vi "Build Measurement.vi"() -> ()   [LabVIEW 2021]
uses:
  <vilib>/Utility/miscctls.llb/LVRowAndColumnTypeDef.ctl
  _Measurement Builder/Measurement Builder/Queue Driver/controls/Queue Operations.ctl
  _Measurement Builder/Measurement Builder/controls/Config File Operations.ctl
  _Measurement Builder/Measurement Builder/controls/Data Holder.ctl
  <vilib>/Utility/miscctls.llb/LVPoint32TypeDef.ctl
  _Measurement Builder/Measurement Builder/controls/Build Spec Details.ctl
  <vilib>/AppBuilder/AB_API_Simple/Get Build Specification Version (path).vi
  _Measurement Builder/Measurement Builder/Queue Driver/Queue Driver.lvlib
  _Measurement Builder/Measurement Builder/Measurement Builder.lvlib
  _Measurement Builder/Measurement Builder/Dictionary/Dictionary.lvlib
  <vilib>/AppBuilder/AB_API_Simple/NI_App_Builder_API.lvlib
panel:
  out "error out":errorcluster
  out "Tab Control":T1(tab)
  in  "Open Directory":bool
  in  "Feed Path":path
  out "Warning":bool=TRUE caption="Feed Path cannot be empty/invalid"
  in  "Next to select":bool
  in  "Build Package":bool
  in  "Project":path caption="LabVIEW Project Path"
  in  "Feed":T2(radio)
  in  "Back 1":bool
  in  "Populate Package":bool
  in  "Select All":bool
  out "Measurement List":i32(listbox)=-1 caption="Select the Measurements to build the package"
  out "Selection warning":string="Selected Project doesn't have EXE build spec"
  out "Maintainer Warning":string
  in  "Settings Page":enum32{"Page 1", "Page 2"}(tab)
  in  "Maintainer Email ID":string="sabthagiri@ni.com"
  in  "Architecture":string(combo)="1"
  in  "Maintainer":string="NI"
  in  "Back 2":bool
  in  "Start Build":bool
  in  "Package List":i32[](listbox) caption="Edit the Package Name and Version"
  in  "Settings":bool
  in  "Progres Bar":i32(slide)=9 caption="Creating Distribution..." scale=0.0..100.0
  in  "Start Next":bool
  in  "Log":bool[](array[boolean])=[TRUE, TRUE]
  in  "Build Status":i32(listbox)=-1
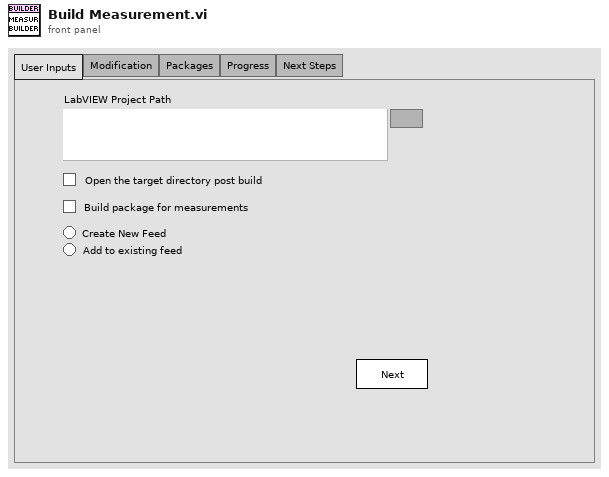
[diagram p1: front panel]
types:
  T1 = enum32{"User Inputs", "Modification", "Packages", "Progress", "Next Steps"}
  T2 = enum32{"No Selection", "CreateFeed", "AddtoFeed"}
  T3 = typedef "Queue Driver.lvlib/Queue Operations.ctl" = enum16{"Create Q", "Enqueue", "Enqueue N", "Dequeue", "Flush", "Release"}
  T4 = typedef "LVRowAndColumnTypeDef.ctl" = cluster{"Row":i32, "Column":i32}
  T5 = enum8{"Enabled", "Disabled", "Disabled and Grayed Out"}
  T6 = typedef "Measurement Builder.lvlib/Config File Operations.ctl" = enum16{"Read", "Write"}
  T7 = typedef "Measurement Builder.lvlib/Data Holder.ctl" = cluster{"Next Clicked?":bool, "MosueDown Coords":T8, "Build Spec":T9[], "No of Meas":i32, "No. of Selected Meas":i32, "Selected Meas":T9[], "Package Details":string[][], "Build Packge?":bool, "Packages Path":path, "Feed":enum32{"No Selection", "CreateFeed", "AddtoFeed"}, "Feed Path":path, "Valid Inputs?":bool, "Feed Old":enum32{"No Selection", "CreateFeed", "AddtoFeed"}, "Status":string[], "Open Directory?":bool}
  T8 = typedef "LVPoint32TypeDef.ctl" = cluster{"Horizontal":i32, "Vertical":i32}
  T9 = typedef "Measurement Builder.lvlib/Build Spec Details.ctl" = cluster{"EXE Name":string, "Target path":path, "Has PPL?":bool, "PPL Name":string}
  T10 = typedef "NI_App_Builder_API.lvlib/Build Specification Version.ctl" = cluster{"Major":u16, "Minor":u16, "Fix":u16, "Build":u16}
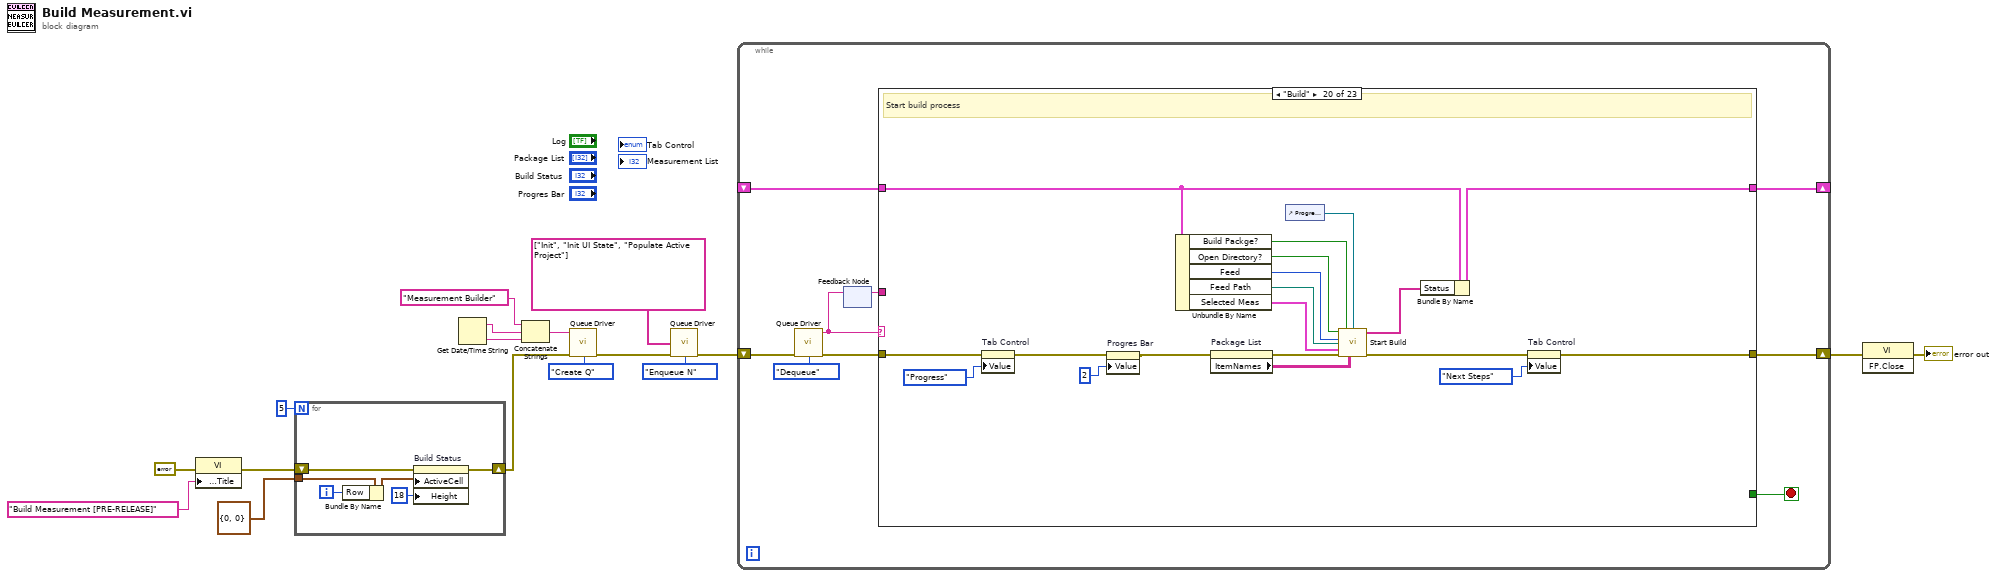
[diagram p0: block diagram]
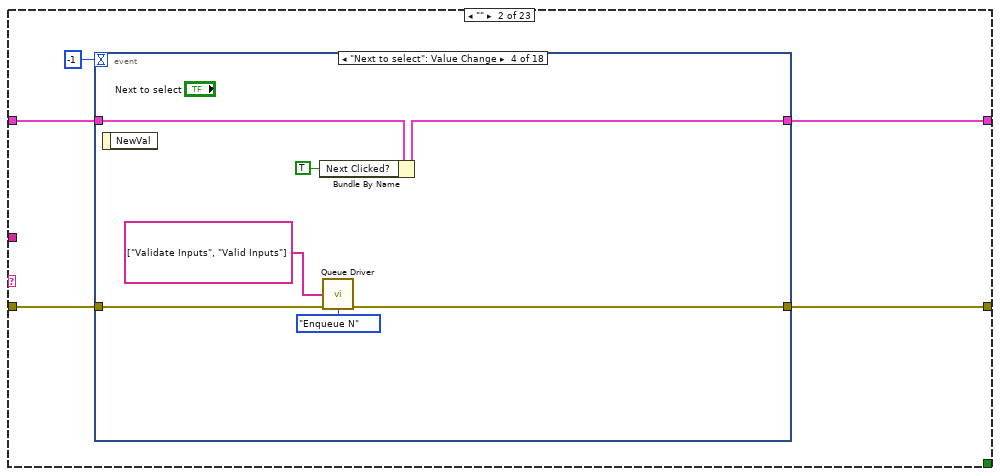
[diagram p3: hidden frame]
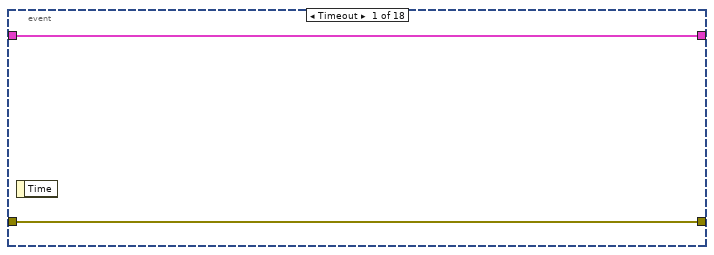
[diagram p4: hidden frame]
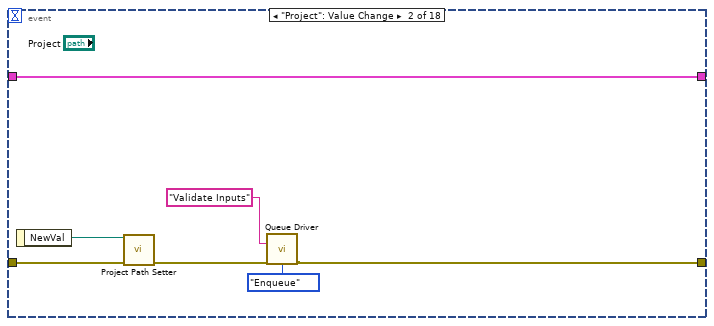
[diagram p5: hidden frame]
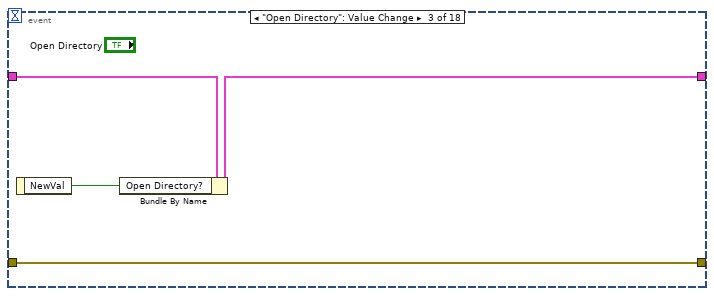
[diagram p6: hidden frame]
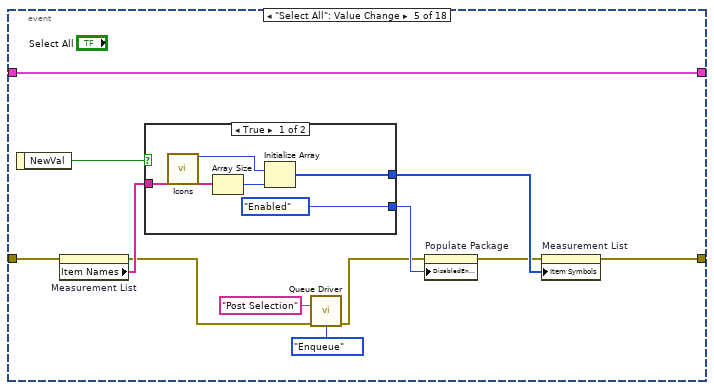
[diagram p7: hidden frame]
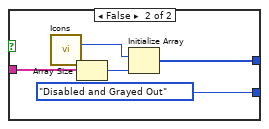
[diagram p8: hidden frame]
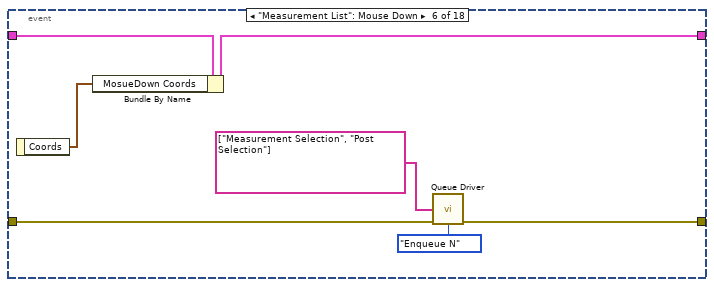
[diagram p9: hidden frame]
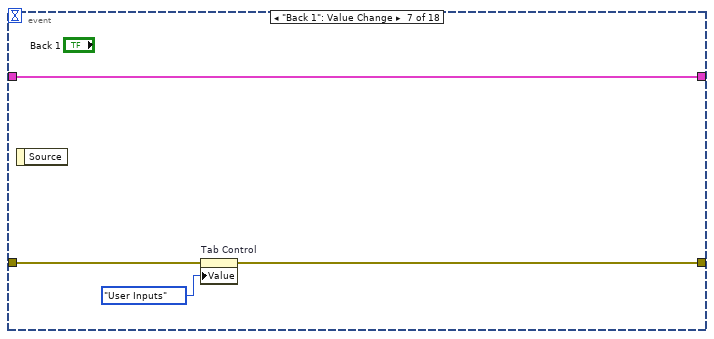
[diagram p10: hidden frame]
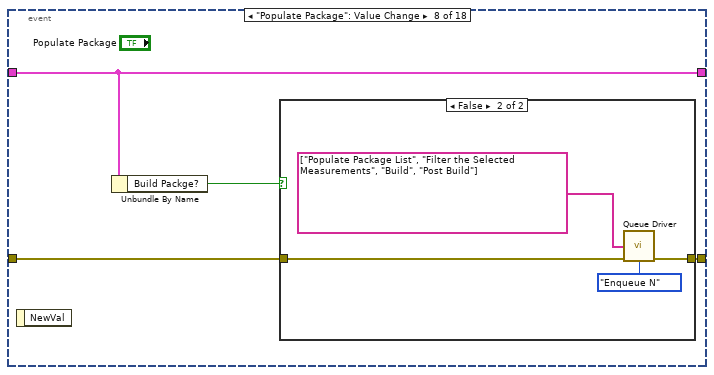
[diagram p11: hidden frame]
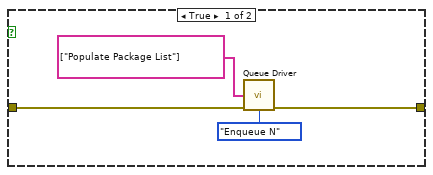
[diagram p12: hidden frame]
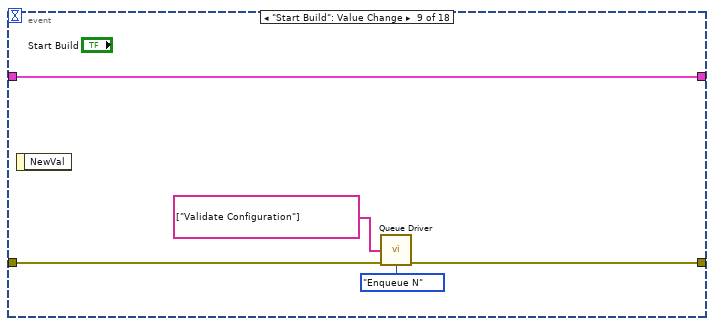
[diagram p13: hidden frame]
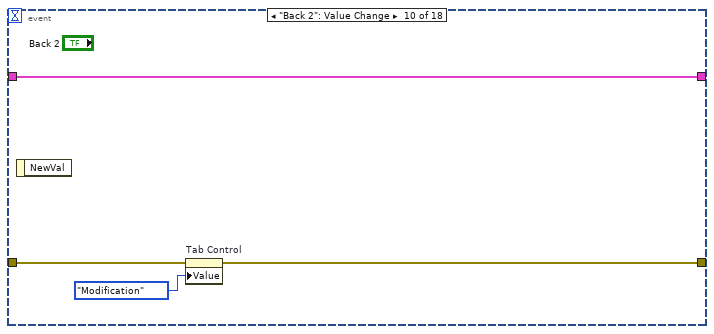
[diagram p14: hidden frame]
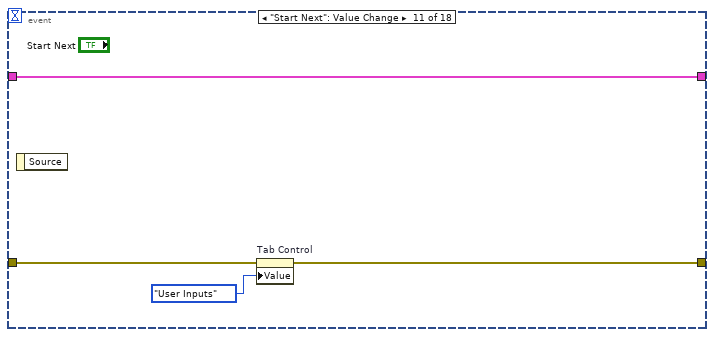
[diagram p15: hidden frame]
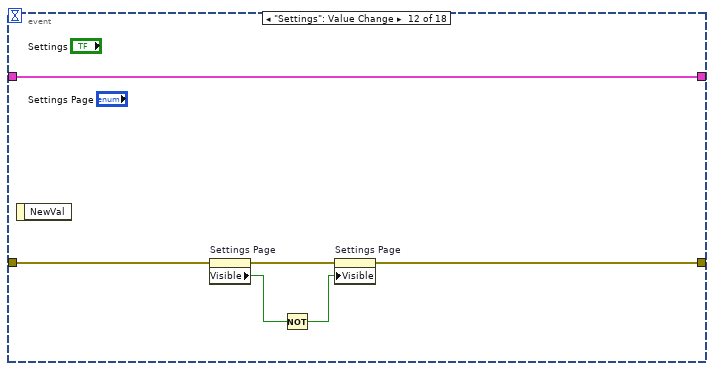
[diagram p16: hidden frame]
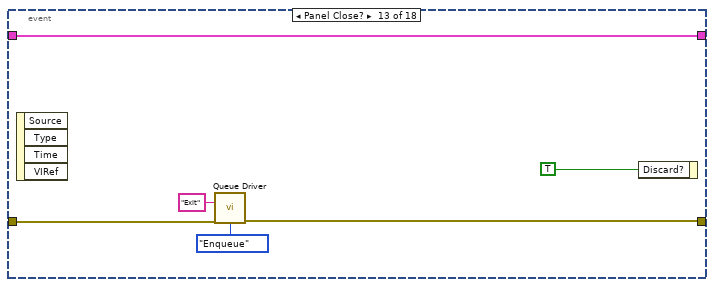
[diagram p17: hidden frame]
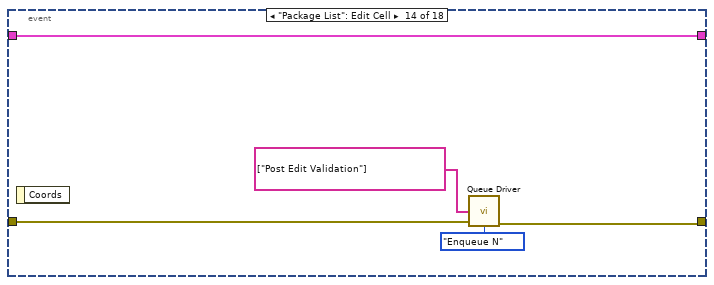
[diagram p18: hidden frame]
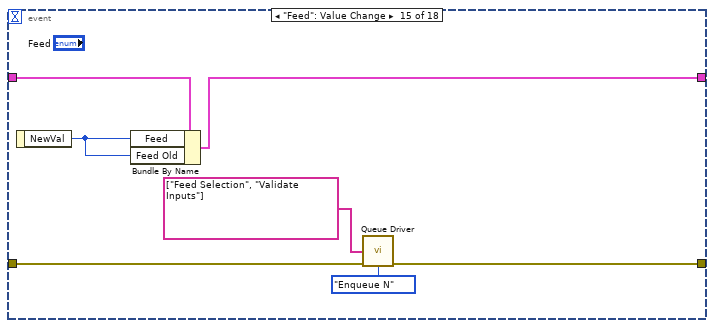
[diagram p19: hidden frame]
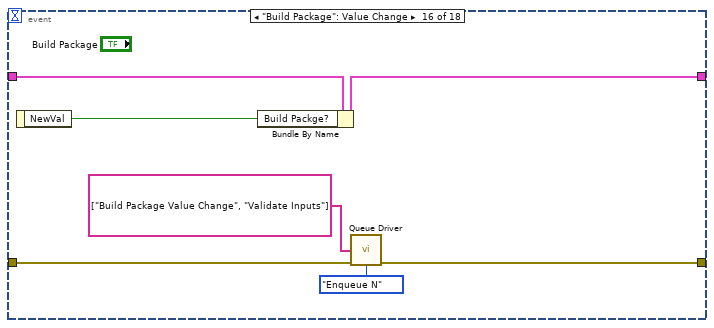
[diagram p20: hidden frame]
diagram:
  n1 = property class="VI"(error in=errorcluster {"status"=FALSE, "code"=0, "source"=""} ("error in (no error)"), "Front Panel.Title"="Build Measurement [PRE-RELEASE]" ("Front Panel Window:Title")) -> (error out=w3:errorcluster)  [unwired: 1 in, 1 out]
  n2 = for {
    N: 5 -> [_]
    tunnel: T4 {"Row"=0, "Column"=0} ("Active Cell:Active Cell") -> [w23]
    shift-right: [w19] -> w6
    shift-left: w3 -> [w18]
    i -> [w21]
    n3 = Bundle By Name(cluster=w23, "Row"=w21) -> (w22:T4)
    n4 = property on="Build Status" class="MCListbox (strict)"(error in=w18, "ActiveCell"=w22, "Height"=u32 18 ("Active Cell:Cell Size:Height")) -> (error out=w19:errorcluster)  [unwired: 1 in, 1 out]
  }
  n5 = Get Date/Time String() -> (date string=w9:string, time string=w10:string)  [unwired: 3 in]
  n6 = Concatenate Strings("Measurement Builder" ("string"), w9, w10) -> (w7:string)
  n7 = call "Queue Driver.vi"("Name"=w7, "error in (no error)"=w6, "Q Operations"=Queue_Operations."Create Q") -> ("error out"=w13:errorcluster)  [unwired: 11 in, 1 out]
  n8 = call "Queue Driver.vi"("States[]"=string[] ["Init", "Init UI State", "Populate Active Project"], "error in (no error)"=w13, "Q Operations"=Queue_Operations."Enqueue N") -> ("error out"=w15:errorcluster)  [unwired: 11 in, 1 out]
  n9 = while {
    shift-right: [w29] -> w5
    shift-left: w15 -> [w32]
    shift-right: [w27] -> _
    shift-left: _ -> [w26]
    stop <- w28 stop-if-true
    n10 = call "Queue Driver.vi"("error in (no error)"=w32, "Q Operations"=Queue_Operations."Dequeue") -> ("Dequeued State"=w25:string, "error out"=w30:errorcluster)  [unwired: 12 in]
    n11 = feedback #1() -> (w24:string)  [unwired: 1 in]
    n12 = feedback-in #1(w25) -> ()
    n13 = case shown="\"Build\"" w25 {
      tunnel: w30 -> [w34 w38 w167 w182 w201 w213 w230 w279 w294 w316 w330 w355 w381 w387 w396 w421 w450 w460 w475 w494 w497 w514 w520]
      tunnel: [w34 w39 w164 w176 w194 w212 w227 w278 w297 w314 w326 w347 w376 w388 w393 w415 w449 w456 w466 w495 w503 w513 w519] -> w29
      tunnel: [_ _ _ _ _ _ _ _ _ _ _ _ _ _ _ _ _ _ _ _ _ _ TRUE] -> w28
      tunnel: [w33 w36 w166 w178 w197 w214 w226 w277 w299 w317 w333 w356 w379 w389 w400 w412 w451 w452 w476 w493 w502 w515 w516] -> w27
      tunnel: w26 -> [w33 w35 _ w178 w198 w214 w225 w277 w300 w317 w333 w356 w382 w389 w400 w409 w451 w454 w476 w487 w502 w515 w516]
      tunnel: w24 -> [_ _ _ _ _ _ _ _ _ _ _ _ _ _ _ _ _ _ _ _ _ _ _]
      frame Default {
      }
      frame "" {
        n14 = event shown="[3] \"Next to select\": Value Change" {
          selector: _ -> [_ _ _ _ _ _ _ _ _ _ _ _ _ _ _ _ _ _]
          dyn-events: _ -> [_ _ _ _ _ _ _ _ _ _ _ _ _ _ _ _ _ _]
          timeout: -1 -> [_ _ _ _ _ _ _ _ _ _ _ _ _ _ _ _ _ _]
          tunnel: [w41 w44 w52 w58 w64 w85 w91 w95 w107 w112 w116 w120 w127 w132 w138 w144 w153 w156] -> w39
          tunnel: w38 -> [w41 w48 w52 w59 w69 w87 w92 w96 w108 w113 w117 w121 w128 w130 w137 w143 w152 w157]
          tunnel: [w40 w42 w50 w55 w71 w84 w90 w94 w109 w111 w115 w118 w124 w134 w140 w147 w155 w161] -> w36
          tunnel: w35 -> [w40 w42 w51 w56 w71 w88 w90 w94 w109 w111 w115 w118 w124 w134 w141 w148 w155 w162]
          event Timeout {
            n15 = event-data() -> ()  [unwired: 1 in, 1 out]
          }
          event "Project": Value Change {
            n16 = event-data() -> ("NewVal"=w47:path)  [unwired: 1 in]
            n17 = call "Project Path Setter.vi"("ProjectPath In"=w47, "error in (no error)"=w48) -> ("error out"=w43:errorcluster)  [unwired: 13 in]
            n18 = call "Queue Driver.vi"("State"="Validate Inputs", "error in (no error)"=w43, "Q Operations"=Queue_Operations."Enqueue") -> ("error out"=w44:errorcluster)  [unwired: 11 in, 1 out]
          }
          event "Open Directory": Value Change {
            n19 = event-data() -> ("NewVal"=w49:bool)  [unwired: 1 in]
            n20 = Bundle By Name(cluster=w51, "Open Directory?"=w49) -> (w50:T7)
          }
          event "Next to select": Value Change {
            n21 = event-data() -> ()  [unwired: 1 in, 1 out]
            n22 = Bundle By Name(cluster=w56, "Next Clicked?"=TRUE) -> (w55:T7)
            n23 = call "Queue Driver.vi"("States[]"=string[] ["Validate Inputs", "Valid Inputs"], "error in (no error)"=w59, "Q Operations"=Queue_Operations."Enqueue N") -> ("error out"=w58:errorcluster)  [unwired: 11 in, 1 out]
          }
          event "Select All": Value Change {
            n24 = event-data() -> ("NewVal"=w70:bool)  [unwired: 1 in]
            n25 = property on="Measurement List" class="LstBox (strict)"(error in=w69) -> (error out=w61:errorcluster, "Item Names"=w68:string[])  [unwired: 1 in, 1 out]
            n26 = case shown="True" w70 {
              tunnel: w68 -> [w75 w80]
              tunnel: [w74 w79] -> w67
              tunnel: [T5."Enabled" ("Disabled") T5."Disabled and Grayed Out" ("Disabled")] -> w66
              frame True {
                n27 = call "Icons.vi"() -> ("Selected"=w72:i32)  [unwired: 14 in, 1 out]
                n28 = Array Size(array=w75) -> (size(s)=w76:i32)
                n29 = Initialize Array(w72, w76) -> (w74:i32[])
              }
              frame False {
                n30 = call "Icons.vi"() -> ("Non Selected"=w77:i32)  [unwired: 14 in, 1 out]
                n31 = Array Size(array=w80) -> (size(s)=w81:i32)
                n32 = Initialize Array(w77, w81) -> (w79:i32[])
              }
            }
            n33 = call "Queue Driver.vi"("State"="Post Selection", "error in (no error)"=w61, "Q Operations"=Queue_Operations."Enqueue") -> ("error out"=w60:errorcluster)  [unwired: 11 in, 1 out]
            n34 = property on="Populate Package" class="Bool"(error in=w60, "DisabledEnum"=w66) -> (error out=w65:errorcluster)  [unwired: 1 in, 1 out]
            n35 = property on="Measurement List" class="LstBox (strict)"(error in=w65, "Item Symbols"=w67) -> (error out=w64:errorcluster)  [unwired: 1 in, 1 out]
          }
          event "Measurement List": Mouse Down {
            n36 = event-data() -> ("Coords"=w83:T8)  [unwired: 1 in]
            n37 = Bundle By Name(cluster=w88, "MosueDown Coords"=w83) -> (w84:T7)
            n38 = call "Queue Driver.vi"("States[]"=string[] ["Measurement Selection", "Post Selection"], "error in (no error)"=w87, "Q Operations"=Queue_Operations."Enqueue N") -> ("error out"=w85:errorcluster)  [unwired: 11 in, 1 out]
          }
          event "Back 1": Value Change {
            n39 = event-data() -> ()  [unwired: 1 in, 1 out]
            n40 = property on="Tab Control" class="TabCtl (strict)"(error in=w92, "Value"=T1."User Inputs" ("Tab Control")) -> (error out=w91:errorcluster)  [unwired: 1 in, 1 out]
          }
          event "Populate Package": Value Change {
            n41 = event-data() -> ()  [unwired: 1 in, 1 out]
            n42 = Unbundle By Name(w94) -> ("Build Packge?"=w93:bool)
            n43 = case shown="False" w93 {
              tunnel: w96 -> [w100 w104]
              tunnel: [w99 w103] -> w95
              frame True {
                n44 = call "Queue Driver.vi"("States[]"=string[] ["Populate Package List"], "error in (no error)"=w100, "Q Operations"=Queue_Operations."Enqueue N") -> ("error out"=w99:errorcluster)  [unwired: 11 in, 1 out]
              }
              frame False {
                n45 = call "Queue Driver.vi"("States[]"=string[] ["Populate Package List", "Filter the Selected Measurements", "Build", "Post Build"], "error in (no error)"=w104, "Q Operations"=Queue_Operations."Enqueue N") -> ("error out"=w103:errorcluster)  [unwired: 11 in, 1 out]
              }
            }
          }
          event "Start Build": Value Change {
            n46 = event-data() -> ()  [unwired: 1 in, 1 out]
            n47 = call "Queue Driver.vi"("States[]"=string[] ["Validate Configuration"], "error in (no error)"=w108, "Q Operations"=Queue_Operations."Enqueue N") -> ("error out"=w107:errorcluster)  [unwired: 11 in, 1 out]
          }
          event "Back 2": Value Change {
            n48 = event-data() -> ()  [unwired: 1 in, 1 out]
            n49 = property on="Tab Control" class="TabCtl (strict)"(error in=w113, "Value"=T1."Modification" ("Tab Control")) -> (error out=w112:errorcluster)  [unwired: 1 in, 1 out]
          }
          event "Start Next": Value Change {
            n50 = event-data() -> ()  [unwired: 1 in, 1 out]
            n51 = property on="Tab Control" class="TabCtl (strict)"(error in=w117, "Value"=T1."User Inputs" ("Tab Control")) -> (error out=w116:errorcluster)  [unwired: 1 in, 1 out]
          }
          event "Settings": Value Change {
            n52 = event-data() -> ()  [unwired: 1 in, 1 out]
            n53 = property on="Settings Page" class="TabCtl (strict)"(error in=w121) -> (error out=w119:errorcluster, "Visible"=w123:bool)  [unwired: 1 in, 1 out]
            n54 = Not(x=w123) -> (.not. x?=w122:bool)
            n55 = property on="Settings Page" class="TabCtl (strict)"(error in=w119, "Visible"=w122) -> (error out=w120:errorcluster)  [unwired: 1 in, 1 out]
          }
          event Panel Close? {
            n56 = event-data() -> ()  [unwired: 1 in, 4 out]
            n57 = call "Queue Driver.vi"("State"="Exit", "error in (no error)"=w128, "Q Operations"=Queue_Operations."Enqueue") -> ("error out"=w127:errorcluster)  [unwired: 11 in, 1 out]
            n58 = event-data("Discard?"=TRUE) -> ()  [unwired: 1 in, 1 out]
          }
          event "Package List": Edit Cell {
            n59 = event-data() -> ()  [unwired: 1 in, 1 out]
            n60 = call "Queue Driver.vi"("States[]"=string[] ["Post Edit Validation"], "error in (no error)"=w130, "Q Operations"=Queue_Operations."Enqueue N") -> ("error out"=w132:errorcluster)  [unwired: 11 in, 1 out]
          }
          event "Feed": Value Change {
            n61 = event-data() -> ("NewVal"=w135:T2)  [unwired: 1 in]
            n62 = Bundle By Name(cluster=w141, "Feed"=w135, "Feed Old"=w135) -> (w140:T7)
            n63 = call "Queue Driver.vi"("States[]"=string[] ["Feed Selection", "Validate Inputs"], "error in (no error)"=w137, "Q Operations"=Queue_Operations."Enqueue N") -> ("error out"=w138:errorcluster)  [unwired: 11 in, 1 out]
          }
          event "Build Package": Value Change {
            n64 = event-data() -> ("NewVal"=w146:bool)  [unwired: 1 in]
            n65 = Bundle By Name(cluster=w148, "Build Packge?"=w146) -> (w147:T7)
            n66 = call "Queue Driver.vi"("States[]"=string[] ["Build Package Value Change", "Validate Inputs"], "error in (no error)"=w143, "Q Operations"=Queue_Operations."Enqueue N") -> ("error out"=w144:errorcluster)  [unwired: 11 in, 1 out]
          }
          event "Architecture", "Maintainer", "Maintainer Email ID": Value Change {
            n67 = event-data() -> ()  [unwired: 1 in, 1 out]
            n68 = call "Read or Write Configurations.vi"("Architecture"="Architecture", "Maintainer"="Maintainer", "Email"="Maintainer Email ID", "error in (no error)"=w152, "Operation"=Config_File_Operations."Write") -> ("error out"=w153:errorcluster)  [unwired: 7 in, 3 out]
          }
          event "Feed Path": Value Change {
            n69 = event-data() -> ("NewVal"=w160:path)  [unwired: 1 in]
            n70 = Bundle By Name(cluster=w162, "Feed Path"=w160) -> (w161:T7)
            n71 = call "Queue Driver.vi"("States[]"=string[] ["Validate Inputs"], "error in (no error)"=w157, "Q Operations"=Queue_Operations."Enqueue N") -> ("error out"=w156:errorcluster)  [unwired: 11 in, 1 out]
          }
        }
      }
      frame "Init" {
        w165 = TRUE ("Open Directory?")
        n72 = invoke class="VI" method="Default Vals.Reinit All"(error in=w167) -> (error out=w163:errorcluster)  [unwired: 2 in, 2 out]
        n73 = property on="Open Directory" class="Bool (strict)"(error in=w163, "Value"=w165) -> (error out=w164:errorcluster)  [unwired: 1 in, 1 out]
        n74 = Bundle By Name(cluster=T7 {"Next Clicked?"=TRUE, "MosueDown Coords"={"Horizontal"=0, "Vertical"=0}, "Build Spec"=[], "No of Meas"=0, "No. of Selected Meas"=0, "Selected Meas"=[], "Package Details"=[], "Build Packge?"=FALSE, "Packages Path"=path "", "Feed"=enum."No Selection", "Feed Path"=path "", "Valid Inputs?"=FALSE, "Feed Old"=enum."No Selection", "Status"=[], "Open Directory?"=FALSE}, "Open Directory?"=w165) -> (w166:T7)
      }
      frame "Init UI State" {
        w175 = u32 16448250 ("Selection Color")
        w172 = FALSE ("Visible")
        n75 = property on="Tab Control" class="TabCtl (strict)"(error in=w182, "Value"=T1."User Inputs" ("Tab Control")) -> (error out=w185:errorcluster)  [unwired: 1 in, 1 out]
        n76 = property on="Settings Page" class="TabCtl (strict)"(error in=w185, "Visible"=w172) -> (error out=w184:errorcluster)  [unwired: 1 in, 1 out]
        n77 = property on="Warning" class="Bool"(error in=w184, "Visible"=w172) -> (error out=w169:errorcluster)  [unwired: 1 in, 1 out]
        n78 = property on="Selection warning" class="Str"(error in=w169, "Visible"=w172) -> (error out=w174:errorcluster)  [unwired: 1 in, 1 out]
        n79 = property on="Feed Path" class="Path"(error in=w174, "Visible"=w172) -> (error out=w173:errorcluster)  [unwired: 1 in, 1 out]
        n80 = property on="Settings" class="Bool"(error in=w173, "Visible"=w172) -> (error out=w171:errorcluster)  [unwired: 1 in, 1 out]
        n81 = property on="Measurement List" class="LstBox (strict)"(error in=w171, "SelColor"=w175) -> (error out=w183:errorcluster)  [unwired: 1 in, 1 out]
        n82 = property on="Package List" class="MCListbox (strict)"(error in=w183, "SelColor"=w175) -> (error out=w177:errorcluster)  [unwired: 1 in, 1 out]
        n83 = property on="Build Status" class="MCListbox (strict)"(error in=w177, "SelColor"=w175) -> (error out=w176:errorcluster)  [unwired: 1 in, 1 out]
        "Selection warning" <- "Atleast one measurement should be selected" ("Selection warning")
        "Maintainer Warning" <- "Maintainer and Email ID cannot be empty" ("Maintainer Warning")
        "Warning" <- TRUE ("Warning")
      }
      frame "Populate Active Project" {
        # "Get the active labview project"
        n84 = call "Get Active ProjectPath.vi"("error in (no error)"=w201) -> ("Project Path"=w189:path, "error out"=w200:errorcluster)  [unwired: 13 in]
        n85 = property on="Project" class="Path"(error in=w200, "Value"=w189) -> (error out=w199:errorcluster)  [unwired: 1 in, 1 out]
        n86 = call "Project Path Setter.vi"("ProjectPath In"=w189, "error in (no error)"=w199) -> ("error out"=w196:errorcluster)  [unwired: 13 in]
        n87 = Empty String/Path?(string/path=w189) -> (empty?=w188:bool)
        n88 = Not A Number/Path/Refnum?(number/path/refnum=w189) -> (NaN/Path/Refnum?=w187:bool)
        n89 = Or(x=w187, y=w188) -> (x .or. y?=w186:bool)
        n90 = case "Not a valid path?" shown="False" w186 {
          tunnel: w198 -> [w206 w211]
          tunnel: [w205 w210] -> w197
          tunnel: [w203 w209] -> w195
          tunnel: [T5."Disabled and Grayed Out" ("Disabled") T5."Enabled" ("Disabled")] -> w192
          frame True {
            w203 = T2."No Selection" ("Feed")
            n91 = Bundle By Name(cluster=w206, "Build Packge?"=FALSE, "Feed"=w203) -> (w205:T7)
          }
          frame False {
            w209 = T2."CreateFeed" ("Feed")
            n92 = Bundle By Name(cluster=w211, "Build Packge?"=TRUE, "Feed"=w209) -> (w210:T7)
          }
        }
        n93 = Not(x=w186) -> (.not. x?=w193:bool)
        n94 = property on="Build Package" class="Bool (strict)"(error in=w196, "Value"=w193) -> (error out=w191:errorcluster)  [unwired: 1 in, 1 out]
        n95 = property on="Feed" class="RadioBtnsControl (strict)"(error in=w191, "DisabledEnum"=w192) -> (error out=w190:errorcluster)  [unwired: 1 in, 1 out]
        n96 = property on="Feed" class="RadioBtnsControl (strict)"(error in=w190, "Value"=w195) -> (error out=w194:errorcluster)  [unwired: 1 in, 1 out]
      }
      frame "Populate Config" {
        # "Disabling it because the config will not be populated in UI"
        # "Populate Config Data"
        n97 = disable-structure shown="Disabled" {
          disable-tunnel: w213 -> [w223 w224]
          disable-tunnel: [w215 w224] -> w212
          frame Disabled {
            n98 = call "Read or Write Configurations.vi"("error in (no error)"=w223, "Operation"=Config_File_Operations."Read") -> ("Architecture OUT"=w221:string, "Maintainer OUT"=w220:string, "Email OUT"=w219:string, "error out"=w218:errorcluster)  [unwired: 10 in]
            n99 = property on="Maintainer Email ID" class="Str"(error in=w218, "Value"=w219) -> (error out=w217:errorcluster)  [unwired: 1 in, 1 out]
            n100 = property on="Maintainer" class="Str"(error in=w217, "Value"=w220) -> (error out=w216:errorcluster)  [unwired: 1 in, 1 out]
            n101 = property on="Architecture" class="CmbBox"(error in=w216, "Value"=w221) -> (error out=w215:errorcluster)  [unwired: 1 in, 1 out]
          }
          frame Enabled {
          }
        }
      }
      frame "Validate Inputs" {
        # "Validate Inputs"
        n102 = call "Validate Project Path.vi"("error in (no error)"=w230) -> ("Valid Path?"=w229:bool, "error out"=w228:errorcluster)  [unwired: 13 in]
        n103 = case "Valid project?" shown="False" w229 {
          tunnel: w228 -> [w236 w244]
          tunnel: [w235 w239] -> w227
          tunnel: [w232 w240] -> w226
          tunnel: w225 -> [w233 w241]
          frame False {
            n104 = property on="Warning" class="Bool"(error in=w236, "Visible"=TRUE, "Caption.Text"="Existing LabVIEW Project Path should be selected" ("Boolean Text.Text")) -> (error out=w235:errorcluster)  [unwired: 1 in, 1 out]
            n105 = Bundle By Name(cluster=w233, "Valid Inputs?"=FALSE) -> (w232:T7)
          }
          frame True {
            n106 = Unbundle By Name(w241) -> ("Build Packge?"=w238:bool, "Feed"=w243:T2, "Feed Path"=w242:path)
            n107 = case "Build package ?" shown="True" w238 {
              tunnel: w244 -> [w246 w256]
              tunnel: w243 -> [_ w255]
              tunnel: w242 -> [_ w254]
              tunnel: w241 -> [w249 w253]
              tunnel: [w248 w252] -> w240
              tunnel: [w250 w251] -> w239
              frame False {
                # "Invalid project Path"
                n108 = Bundle By Name(cluster=w249, "Valid Inputs?"=TRUE) -> (w248:T7)
                n109 = property on="Warning" class="Bool"(error in=w246, "Visible"=FALSE) -> (error out=w250:errorcluster)  [unwired: 1 in, 1 out]
              }
              frame True {
                n110 = case shown="Default" w255 {
                  tunnel: w256 -> [w263 w271]
                  tunnel: w254 -> [w264 _]
                  tunnel: w253 -> [w269 w275]
                  tunnel: [w268 w274] -> w252
                  tunnel: [w266 w270] -> w251
                  frame "AddtoFeed" {
                    # "Validate Path"
                    n111 = Empty String/Path?(string/path=w264) -> (empty?=w262:bool)
                    n112 = call <vilib>:"Check if File or Folder Exists.vi"("error in (no error)"=w263, "path"=w264) -> ("error out"=w258:errorcluster, "file or folder exists?"=w260:bool)  [unwired: 7 in, 1 out]
                    n113 = Not A Number/Path/Refnum?(number/path/refnum=w264) -> (NaN/Path/Refnum?=w261:bool)
                    n114 = Or(x=w262, y=w261) -> ()  [unwired: 1 out]
                    n115 = Not(x=w260) -> (.not. x?=w257:bool)
                    n116 = Compound Arithmetic op=OR(w262, w261, w257) -> (w259:bool)
                    n117 = Not(x=w259) -> (.not. x?=w265:bool)
                    n118 = Bundle By Name(cluster=w269, "Valid Inputs?"=w265) -> (w268:T7)
                    n119 = property on="Warning" class="Bool"(error in=w258, "Visible"=w259, "Caption.Text"="Feed Path cannot be empty/invalid" ("Boolean Text.Text")) -> (error out=w266:errorcluster)  [unwired: 1 in, 1 out]
                  }
                  frame Default {
                    n120 = property on="Warning" class="Bool"(error in=w271, "Visible"=FALSE) -> (error out=w270:errorcluster)  [unwired: 1 in, 1 out]
                    n121 = Bundle By Name(cluster=w275, "Valid Inputs?"=TRUE) -> (w274:T7)
                  }
                }
              }
            }
          }
        }
      }
      frame "Valid Inputs" {
        # "Check if valid inputs and if next is clicked"
        n122 = Unbundle By Name(w277) -> ("Valid Inputs?"=w276:bool)
        n123 = case "Valid Inputs?" shown="True" w276 {
          tunnel: w279 -> [w280 w286]
          tunnel: [w280 w282] -> w278
          tunnel: w277 -> [_ w281]
          frame False {
          }
          frame True {
            n124 = Unbundle By Name(w281) -> ("Next Clicked?"=w283:bool)
            n125 = property on="Warning" class="Bool"(error in=w286, "Visible"=FALSE) -> (error out=w284:errorcluster)  [unwired: 1 in, 1 out]
            n126 = case "Next Clicked?" shown="True" w283 {
              tunnel: w284 -> [w287 w290]
              tunnel: [w287 w288] -> w282
              frame False {
              }
              frame True {
                n127 = call "Queue Driver.vi"("States[]"=string[] ["Populate Measurements", "Update Tab", "Validate Measurement"], "error in (no error)"=w290, "Q Operations"=Queue_Operations."Enqueue N") -> ("error out"=w288:errorcluster)  [unwired: 11 in, 1 out]
              }
            }
          }
        }
      }
      frame "Build Package Value Change" {
        # "Build Package Value Change Handling"
        n128 = Unbundle By Name(w300) -> ("Feed"=w293:T2, "Build Packge?"=w301:bool, "Feed Old"=w296:T2)
        n129 = case shown="False" w301 {
          tunnel: w300 -> [w306 w312]
          tunnel: [w305 w309] -> w299
          tunnel: [T5."Disabled and Grayed Out" ("Disabled") T5."Enabled" ("Disabled")] -> w302
          tunnel: w296 -> [w303 w308]
          tunnel: [_ w310] -> w295
          tunnel: w293 -> [w304 _]
          tunnel: [w303 w308] -> w292
          frame False {
            n130 = Bundle By Name(cluster=w306, "Feed Old"=w304) -> (w305:T7)
          }
          frame True {
            n131 = case shown="\"AddtoFeed\"" w308 {
              tunnel: [TRUE _] -> w310
              frame "AddtoFeed" {
              }
              frame Default {
              }
            }
            n132 = Bundle By Name(cluster=w312, "Feed"=w308) -> (w309:T7)
          }
        }
        n133 = property on="Feed Path" class="Path"(error in=w294, "Visible"=w295) -> (error out=w298:errorcluster)  [unwired: 1 in, 1 out]
        n134 = property on="Feed" class="RadioBtnsControl (strict)"(error in=w298, "DisabledEnum"=w302, "Value"=w292) -> (error out=w297:errorcluster)  [unwired: 1 in, 1 out]
      }
      frame "Feed Selection" {
        # "Feed Selection Value Change Handling"
        n135 = Unbundle By Name(w317) -> ("Feed"=w315:T2)
        n136 = case shown="Default" w315 {
          tunnel: w316 -> [w319 w323]
          tunnel: [w318 w321] -> w314
          frame Default {
            n137 = property on="Feed Path" class="Path"(error in=w319, "Visible"=FALSE) -> (error out=w318:errorcluster)  [unwired: 1 in, 1 out]
          }
          frame "AddtoFeed" {
            n138 = property on="Feed Path" class="Path"(error in=w323, "Visible"=TRUE) -> (error out=w321:errorcluster)  [unwired: 1 in, 1 out]
          }
        }
      }
      frame "Measurement Selection" {
        # "Measurement Selection Value change"
        n139 = Unbundle By Name(w333) -> ("No of Meas"=w324:i32, "MosueDown Coords"=w332:T8)
        n140 = property on="Measurement List" class="LstBox (strict)"(error in=w330) -> (error out=w329:errorcluster, "Item Symbols"=w327:i32[])  [unwired: 1 in, 1 out]
        n141 = invoke on="Measurement List" class="LstBox (strict)" method="Point To Row"(error in=w329, "Point"=w332) -> (error out=w331:errorcluster, "Row"=w325:i32)  [unwired: 5 in, 5 out]
        n142 = Greater?(x=w324, y=w325) -> (0:w328:bool)
        n143 = case "Mouse click In range?" shown="True" w328 {
          tunnel: w331 -> [w334 w337]
          tunnel: w327 -> [_ w339]
          tunnel: [w334 w336] -> w326
          tunnel: w325 -> [_ w335]
          frame False {
          }
          frame True {
            # "Change the item symbols"
            n144 = in-place {
              n145 = in-place-array #2(w339, w335) -> (w343:i32)
              n146 = call "Icons.vi"() -> ("Selected"=w342:i32, "Non Selected"=w344:i32)  [unwired: 14 in]
              n147 = Equal?(x=w343, y=w342) -> (x = y?=w341:bool)
              n148 = Swap Values(12:w342, 13:w341, 14:w344) -> (1:w340:i32)  [unwired: 1 out]
              n149 = in-place-array #2(w340) -> (w338:i32[])  [unwired: 1 out]
            }
            n150 = property on="Measurement List" class="LstBox (strict)"(error in=w337, "Item Symbols"=w338) -> (error out=w336:errorcluster)  [unwired: 1 in, 1 out]
          }
        }
      }
      frame "Post Selection" {
        # "Selection change handling"
        n151 = property on="Measurement List" class="LstBox (strict)"(error in=w355) -> (error out=w352:errorcluster, "Item Symbols"=w354:i32[])  [unwired: 1 in, 1 out]
        n152 = call "Check the Symbols.vi"("Item Symbols"=w354) -> ("All Selected?"=w353:bool, "None Selected"=w351:bool)  [unwired: 13 in]
        n153 = case "All selected?" shown="False" w353 {
          tunnel: w352 -> [w360 w372]
          tunnel: w351 -> [w363 _]
          tunnel: [w361 T5."Enabled" ("Disabled")] -> w350
          tunnel: [w359 w369] -> w349
          tunnel: [w357 _] -> w346
          frame False {
            n154 = property on="Select All" class="Bool (strict)"(error in=w360, "Value"=FALSE ("All")) -> (error out=w358:errorcluster)  [unwired: 1 in, 1 out]
            n155 = case "None Selected?" shown="False" w363 {
              tunnel: [T5."Enabled" ("Disabled") T5."Disabled and Grayed Out" ("Disabled")] -> w361
              tunnel: [w364 w367] -> w359
              tunnel: w358 -> [w364 w367]
              tunnel: [_ TRUE] -> w357
              frame False {
              }
              frame True {
              }
            }
          }
          frame True {
            n156 = property on="Select All" class="Bool (strict)"(error in=w372, "Value"=TRUE ("All")) -> (error out=w369:errorcluster)  [unwired: 1 in, 1 out]
          }
        }
        n157 = property on="Populate Package" class="Bool"(error in=w349, "DisabledEnum"=w350) -> (error out=w348:errorcluster)  [unwired: 1 in, 1 out]
        n158 = property on="Selection warning" class="Str"(error in=w348, "Visible"=w346, "Value"="Atleast one measurement should be selected" ("Selection warning")) -> (error out=w347:errorcluster)  [unwired: 1 in, 1 out]
      }
      frame "Populate Measurements" {
        # "Populate the selected measurements with the package name"
        n159 = call "Get Measurement Names.vi"("error in (no error)"=w381) -> ("Build Details"=w378:T9[], "error out"=w380:errorcluster)  [unwired: 13 in]
        n160 = for {
          tunnel: w378 -> [w385] mode=indexing
          tunnel: [w384] -> w374 mode=indexing
          tunnel: [w383] -> w377 mode=indexing
          n161 = Unbundle By Name(w385) -> ("EXE Name"=w384:string)
          n162 = call "Icons.vi"() -> ("Selected"=w383:i32)  [unwired: 14 in, 1 out]
        }
        n163 = property on="Measurement List" class="LstBox (strict)"(error in=w380, "Item Names"=w374, "Item Symbols"=w377, "Active Row"=-1 ("Selection Mode")) -> (error out=w376:errorcluster)  [unwired: 1 in, 1 out]
        n164 = Array Size(array=w374) -> (size(s)=w373:i32)
        n165 = Bundle By Name(cluster=w382, "Build Spec"=w378, "No of Meas"=w373, "No. of Selected Meas"=w373) -> (w379:T7)
      }
      frame "Update Tab" {
        n166 = property on="Tab Control" class="TabCtl (strict)"(error in=w387, "Value"=T1."Modification" ("Tab Control")) -> (error out=w388:errorcluster)  [unwired: 1 in, 1 out]
      }
      frame "Validate Measurement" {
        # "Validate measurements"
        n167 = Unbundle By Name(w400) -> ("Build Spec"=w399:T9[])
        n168 = Empty Array?(array=w399) -> (empty?=w398:bool)
        n169 = case shown="False" w398 {
          tunnel: [T5."Enabled" ("Disabled") T5."Disabled and Grayed Out" ("Disabled")] -> w397
          tunnel: [TRUE ("All") FALSE ("All")] -> w392
          frame False {
          }
          frame True {
          }
        }
        n170 = property on="Populate Package" class="Bool"(error in=w396, "DisabledEnum"=w397) -> (error out=w395:errorcluster)  [unwired: 1 in, 1 out]
        n171 = property on="Select All" class="Bool (strict)"(error in=w395, "Value"=w392, "DisabledEnum"=w397) -> (error out=w394:errorcluster)  [unwired: 1 in, 1 out]
        n172 = Not(x=w392) -> (.not. x?=w391:bool)
        n173 = property on="Selection warning" class="Str"(error in=w394, "Visible"=w391, "Value"="Selected Project doesn't have EXE build spec" ("Selection warning")) -> (error out=w393:errorcluster)  [unwired: 1 in, 1 out]
      }
      frame "Populate Package List" {
        # "Populate Package List"
        n174 = property on="Measurement List" class="LstBox (strict)"(error in=w421) -> (error out=w408:errorcluster, "Item Names"=w420:string[], "Item Symbols"=w419:i32[])  [unwired: 1 in, 1 out]
        n175 = call "Project Path Getter.vi"("error in (no error)"=w408) -> ("Path"=w406:path, "error out"=w407:errorcluster)  [unwired: 13 in]
        n176 = for {
          tunnel: w420 -> [w425] mode=indexing
          tunnel: w419 -> [w429] mode=indexing
          tunnel: [w425] -> w418 mode=indexing if=w424
          tunnel: [w428] -> w410 mode=indexing if=w424
          shift-right: [w426] -> w417
          shift-left: w407 -> [w427]
          tunnel: w406 -> [w422]
          n177 = call "Icons.vi"() -> ("Selected"=w423:i32)  [unwired: 14 in, 1 out]
          n178 = Equal?(x=w429, y=w423) -> (x = y?=w424:bool)
          n179 = case shown="True" w424 {
            tunnel: [_ w437] -> w428
            tunnel: w427 -> [w430 w442]
            tunnel: [w430 w439] -> w426
            tunnel: w425 -> [_ w443]
            tunnel: w422 -> [_ w441]
            frame False {
            }
            frame True {
              n180 = call-poly <vilib>:"Get Build Specification Version.vi"("error in (no error)"=w442, "Name of build specification"=w443, "Path to project"=w441) -> ("error out"=w438:errorcluster, "Build Specification Version"=w432:T10)  [unwired: 7 in]
              n181 = call "Check Initial Version.vi"("Build Version In"=w432) -> ("Build Version Out"=w431:T10)  [unwired: 14 in]
              n182 = Unbundle By Name(w431) -> ("Major"=w436:u16, "Minor"=w435:u16, "Fix"=w434:u16, "Build"=w433:u16)
              n183 = Format Into String(format string="%d.%d.%d.%d", error in=w438, w436, w435, w434, w433) -> (resulting string=w437:string, error out=w439:errorcluster)  [unwired: 1 in]
            }
          }
        }
        n184 = Build Array(w418, w410) -> (w414:string[][])
        n185 = Transpose 2D Array(2D array=w414) -> (transposed array=w411:string[][])
        n186 = property on="Package List" class="MCListbox (strict)"(error in=w417, "ItemNames"=w411, "SelMode"=0 ("Selection Mode")) -> (error out=w416:errorcluster)  [unwired: 1 in, 1 out]
        n187 = Bundle By Name(cluster=w409, "Package Details"=w411) -> (w412:T7)
        n188 = property on="Tab Control" class="TabCtl (strict)"(error in=w416, "Value"=T1."Packages" ("Tab Control")) -> (error out=w415:errorcluster)  [unwired: 1 in, 1 out]
      }
      frame "Validate Configuration" {
        w446 = FALSE ("Visible")
        # "Check if configuration maintainer, maintainer email ID is valid"
        n189 = call "Queue Driver.vi"("States[]"=string[] ["Filter the Selected Measurements", "Build", "Post Build"], "error in (no error)"=w450, "Q Operations"=Queue_Operations."Enqueue N") -> ("error out"=w447:errorcluster)  [unwired: 11 in, 1 out]
        n190 = property on="Settings Page" class="TabCtl (strict)"(error in=w447, "Visible"=w446) -> (error out=w445:errorcluster)  [unwired: 1 in, 1 out]
        n191 = property on="Maintainer Warning" class="Str"(error in=w445, "Visible"=w446) -> (error out=w449:errorcluster)  [unwired: 1 in, 1 out]
      }
      frame "Filter the Selected Measurements" {
        # "Get the selected measurements"
        n192 = property on="Measurement List" class="LstBox (strict)"(error in=w460) -> (error out=w457:errorcluster, "Item Names"=w458:string[], "Item Symbols"=w459:i32[])  [unwired: 1 in, 1 out]
        n193 = Unbundle By Name(w454) -> ("Build Spec"=w455:T9[])
        n194 = call "Get Selected Meas Data.vi"("Build Spec"=w455, "Item Names"=w458, "Item Symbols"=w459, "error in (no error)"=w457) -> ("Selected Meas"=w453:T9[], "error out"=w456:errorcluster)  [unwired: 10 in]
        n195 = Bundle By Name(cluster=w454, "Selected Meas"=w453) -> (w452:T7)
      }
      frame "Post Edit Validation" {
        # "After editing validate if the changes are valid"
        n196 = Unbundle By Name(w476) -> ("Package Details"=w474:string[][])
        n197 = property on="Package List" class="MCListbox (strict)"(error in=w475) -> (error out=w468:errorcluster, "ItemNames"=w472:string[][])  [unwired: 1 in, 1 out]
        n198 = Index Array(array=w474, index (col) #1=0 ("disabled index (col)"), index (col) #2=1 ("disabled index (col)")) -> (element #1=w469:string[], element #2=w462:string[])  [unwired: 2 in]
        n199 = Index Array(array=w472, index (col)=1 ("disabled index (col)")) -> (element=w461:string[])  [unwired: 1 in]
        n200 = call "Validate the version.vi"("Old Version"=w462, "New Version"=w461, "error in (no error)"=w468) -> ("Version Out"=w463:string[], "error out"=w467:errorcluster)  [unwired: 11 in]
        n201 = Build Array(w469, w463) -> (w464:string[][])
        n202 = Transpose 2D Array(2D array=w464) -> (transposed array=w465:string[][])
        n203 = property on="Package List" class="MCListbox (strict)"(error in=w467, "ItemNames"=w465) -> (error out=w466:errorcluster)  [unwired: 1 in, 1 out]
      }
      frame "Build" {
        # "Start build process"
        n204 = property on="Tab Control" class="TabCtl (strict)"(error in=w494, "Value"=T1."Progress" ("Tab Control")) -> (error out=w490:errorcluster)  [unwired: 1 in, 1 out]
        n205 = property on="Progres Bar" class="Slide (strict)"(error in=w490, "Value"=2 ("Progres Bar")) -> (error out=w491:errorcluster)  [unwired: 1 in, 1 out]
        n206 = Unbundle By Name(w487) -> ("Build Packge?"=w481:bool, "Open Directory?"=w480:bool, "Feed"=w479:T2, "Feed Path"=w478:path, "Selected Meas"=w477:T9[])
        n207 = property on="Package List" class="MCListbox (strict)"(error in=w491) -> (error out=w486:errorcluster, "ItemNames"=w485:string[][])  [unwired: 1 in, 1 out]
        n208 = control-ref of="Progres Bar"() -> (w482:refnum<vi>)
        n209 = call "Start Build.vi"("Open Directory?"=w480, "Build Packge?"=w481, "Progres Bar"=w482, "Feed"=w479, "Feed Path"=w478, "Selected Meas"=w477, "error in (no error)"=w486, "Package Spec"=w485) -> ("Status"=w483:string[], "error out"=w484:errorcluster)  [unwired: 6 in]
        n210 = Bundle By Name(cluster=w487, "Status"=w483) -> (w493:T7)
        n211 = property on="Tab Control" class="TabCtl (strict)"(error in=w484, "Value"=T1."Next Steps" ("Tab Control")) -> (error out=w495:errorcluster)  [unwired: 1 in, 1 out]
      }
      frame "Post Build" {
        # "Populate the results in post build"
        n212 = Unbundle By Name(w502) -> ("Selected Meas"=w501:T9[], "Status"=w496:string[])
        n213 = for {
          tunnel: w501 -> [w506] mode=indexing
          tunnel: [w505] -> w500 mode=indexing
          tunnel: [""] -> _ mode=indexing
          n214 = Unbundle By Name(w506) -> ("EXE Name"=w505:string)
        }
        n215 = Build Array(w500, w496) -> (w499:string[][])
        n216 = Transpose 2D Array(2D array=w499) -> (transposed array=w498:string[][])
        n217 = property on="Build Status" class="MCListbox (strict)"(error in=w497, "ItemNames"=w498) -> (error out=w503:errorcluster)  [unwired: 1 in, 1 out]
      }
      frame "Error" {
        n218 = call <vilib>:"Simple Error Handler.vi"("error in (no error)"=w514) -> ("error out"=w507:errorcluster)  [unwired: 4 in, 4 out]
        n219 = call <vilib>:"Clear Errors.vi"("error in (no error)"=w507) -> ("error out"=w510:errorcluster)  [unwired: 5 in, 1 out]
        n220 = call "Queue Driver.vi"("error in (no error)"=w510, "Q Operations"=Queue_Operations."Flush") -> ("error out"=w509:errorcluster)  [unwired: 12 in, 1 out]
        n221 = call "Queue Driver.vi"("State"="Exit", "error in (no error)"=w509, "Q Operations"=Queue_Operations."Enqueue") -> ("error out"=w513:errorcluster)  [unwired: 11 in, 1 out]
      }
      frame "Exit" {
        n222 = call "Queue Driver.vi"("error in (no error)"=w520, "Q Operations"=Queue_Operations."Flush") -> ("error out"=w518:errorcluster)  [unwired: 12 in, 1 out]
        n223 = call "Queue Driver.vi"("error in (no error)"=w518, "Q Operations"=Queue_Operations."Release") -> ("error out"=w519:errorcluster)  [unwired: 12 in, 1 out]
      }
    }
  }
  n224 = invoke class="VI" method="FP.Close"(error in=w5) -> (error out=→"error out":errorcluster)  [unwired: 2 in, 2 out]
